vi "Create Sensor.vi"(8 "error in (no error)":errorcluster, 11 "Create Sensor Model in":refnum<class "Create Sensor Model.lvclass">) -> (0 "error out":errorcluster, 3 "Create Sensor Model out":refnum<class "Create Sensor Model.lvclass">)   [LabVIEW 2013, in "Create Sensor Model.lvlib" / "Create Sensor Model.lvclass"]
uses:
  Create Sensor Model.lvclass
  Create Sensor Model.lvclass/Create Sensor Model.ctl
  Common/File IO/File IO.lvlib
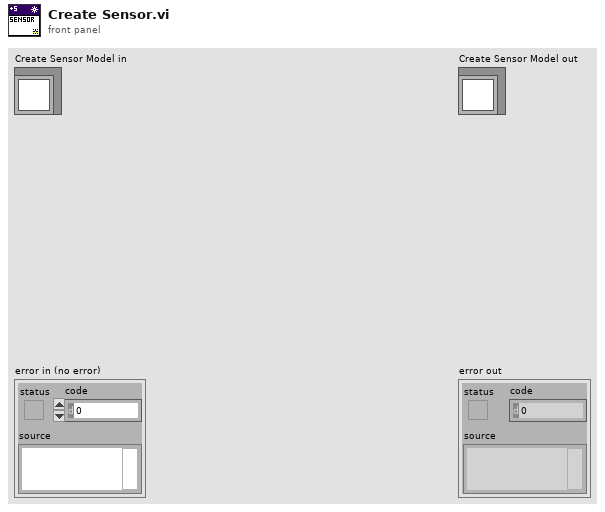
[diagram p1: front panel]
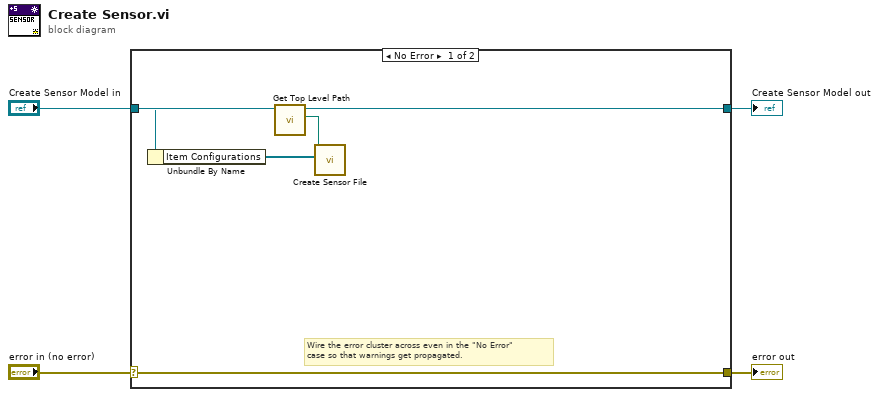
[diagram p0: block diagram]
diagram:
  n1 = case shown="No Error" "error in (no error)" {
    selector: "error in (no error)" -> [w9 w11]
    tunnel: [w9 w11] -> w2
    tunnel: [w7 w10] -> w3
    tunnel: "Create Sensor Model in" -> [w8 w10]
    frame No Error {
      # "Wire the error cluster across even in the \"No Error\"\ncase so that warnings get propagated."
      n2 = call-dynamic "Get Top Level Path.vi"("Abstract Model in"=w8) -> ("Top Level Path"=w6:path, "Abstract Model out"=w7:refnum<class "Create Sensor Model.lvclass">)  [unwired: 8 in, 1 out]
      n3 = Unbundle By Name(w7) -> ("Item Configurations"=w5:refnum<class "Item Configuration.lvclass">[])
      n4 = call "Create Sensor File.vi"("Item Configurations"=w5, "Top Level Path"=w6) -> ()  [unwired: 9 in, 1 out]
    }
    frame Error {
    }
  }
  "error out" <- w2
  "Create Sensor Model out" <- w3
